vi "Label.vi"(8 "error in (no error)":errorcluster, 10 "Label":T1, 11 "ITX Commands in":refnum<class "ITX Commands.lvclass">) -> (0 "error out":errorcluster, 3 "ITX Commands out":refnum<class "ITX Commands.lvclass">)   [LabVIEW 2019, in "ITX Commands.lvclass"]
uses:
  ITX Commands.lvclass
  typedefs/Label--cluster.ctl
  ITX Commands.lvclass/ITX Commands.ctl
panel:
  out "resulting string":string
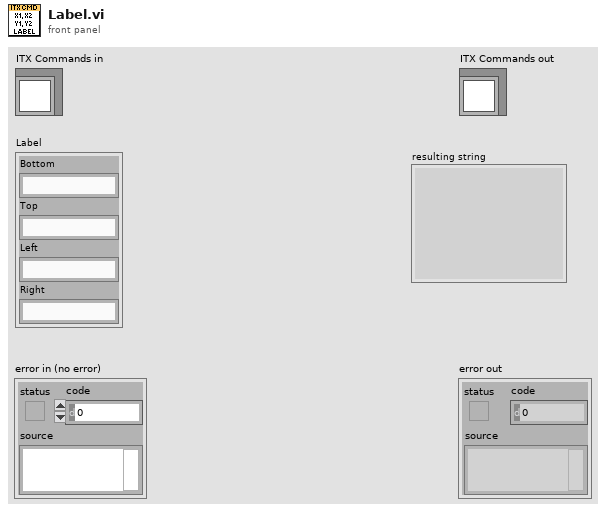
[diagram p1: front panel]
types:
  T1 = typedef "ITX Commands.lvclass/Label--cluster.ctl" = cluster{"Bottom":string, "Top":string, "Left":string, "Right":string}
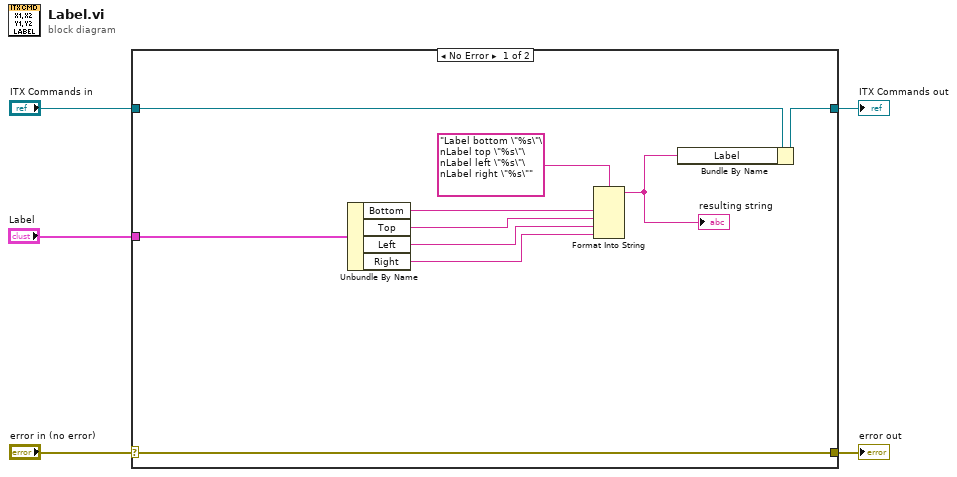
[diagram p0: block diagram]
diagram:
  n1 = case shown="No Error" "error in (no error)" {
    selector: "error in (no error)" -> [w8 w17]
    tunnel: [w8 w17] -> w4
    tunnel: [w9 w16] -> w2
    tunnel: "ITX Commands in" -> [w15 w16]
    tunnel: "Label" -> [w7 _]
    frame No Error {
      n2 = Unbundle By Name(w7) -> ("Bottom"=w13:string, "Top"=w12:string, "Left"=w11:string, "Right"=w10:string)
      n3 = Format Into String(format string="Label bottom \"%s\"\nLabel top \"%s\"\nLabel left \"%s\"\nLabel right \"%s\"", w13, w12, w11, w10) -> (resulting string=w6:string)  [unwired: 2 in, 1 out]
      "resulting string" <- w6
      n4 = Bundle By Name(cluster=w15, "Label"=w6) -> (w9:refnum<class "ITX Commands.lvclass">)
    }
    frame Error {
    }
  }
  "error out" <- w4
  "ITX Commands out" <- w2
